vi "Data Recorder.vi"() -> ()   [LabVIEW 2017]
uses:
  LabVIEW/Controls/Recording Settings.ctl
  LabVIEW/Controls/Operator Settings.ctl
  LabVIEW/Controls/Operator.ctl
  LabVIEW/Controls/Patient Settings.ctl
  LabVIEW/Controls/Refnums.ctl
  LabVIEW/Controls/Dimensions.ctl
  LabVIEW/Controls/Room Dimensions.ctl
  LabVIEW/Controls/Crop Type.ctl
  <vilib>/vision/Image Controls.llb/IMAQ Image.ctl
  LabVIEW/Controls/Rigid Body Info.ctl
  LabVIEW/Controls/Position.ctl
  LabVIEW/Controls/Orientation.ctl
  LabVIEW/Controls/Enabled State Control.ctl
  LabVIEW/Controls/Frame Grabber State.ctl
  LabVIEW/Controls/Optitrack State.ctl
  LabVIEW/Controls/Frame Grabber Data.ctl
  <vilib>/userdefined/High Color/IMAQdx.ctl
  <vilib>/vision/Avi.llb/IMAQ AVI2 Refnum.ctl
  LabVIEW/Controls/Crop Video State.ctl
panel:
  out "Rigid Bodies":T1[](array[typedef])
  out "Mask":T4
  in  "Crop Type":T5
  out "Initial Recording Settings":T6={"Folder to Save Recordings"=path "", "Video FPS"=5, "Codec"=3, "Tracker FPS"=40, "Operator ID"={"Operator ID"=0, "Expertise"=0}, "Patient ID/Gestation"={"ID"=0, "Gestation"=""}} {"Patient ID/Gestation"."ID" format="%0#3.2f"; "Operator ID"."Operator ID" format="%03.0f"; "Operator ID"."Expertise" items=["Novice", "Expert"]; "Tracker FPS" max=100; "Codec" items=["Cinepak Codec by Radius", "Intel IYUV codec", "Microsoft Video 1", "FF Video Codec 1 (FFV1) (NI Vision)", "Motion JPEG (NI Vision)", "Y800 Uncompressed Grey Scale (NI Vision)", "YUV 4:2:0 Planar (NI Vision)"]; "Video FPS" max=100}
  in  "Dimensions":T10={"Probe Dimensions"={"Probe Width"=50.0, "Probe Depth"=100.0, "Probe Height"=150.0}, "Room Dimensions"={"Room Width"=1000.0, "Room Depth"=1000.0, "Room Height"=1000.0}}
  in  "Playback Rate":dbl(knob)=10.0 min=1.0 max=100.0 scale=1.0..100.0
  out "Time (s)":dbl caption="s"
  in  "Refnums":T12
  out "Tracked?":bool
  out "Crop ROI":i32[](array[numeric])
  in  "Clear Crop":bool
  in  "Append":bool
  in  "Presentation":string
  in  "Crop":bool
  in  "Pause":bool
  out "Video Playback Filename":path=path "C:/Users/lydia/Desktop/Images/Breech_Sacro_Posterior-20191119160600.avi"
  in  "Frame Slider":u32(slide)=175 scale=0.0..8635370.0
  in  "Playback":bool
  in  "Home":bool
  in  "Recording Settings":T6={"Folder to Save Recordings"=path "C:/Users/lydia/Desktop/Images", "Video FPS"=5, "Codec"=3, "Tracker FPS"=40, "Operator ID"={"Operator ID"=0, "Expertise"=0}, "Patient ID/Gestation"={"ID"=0, "Gestation"=""}} {"Patient ID/Gestation"."ID" format="%0#3.2f"; "Operator ID"."Operator ID" format="%03.0f"; "Operator ID"."Expertise" items=["Novice", "Expert"]; "Codec" items=["Cinepak Codec by Radius", "Intel IYUV codec", "Microsoft Video 1", "FF Video Codec 1 (FFV1) (NI Vision)", "Motion JPEG (NI Vision)", "Y800 Uncompressed Grey Scale (NI Vision)", "YUV 4:2:0 Planar (NI Vision)"]; "Video FPS" max=100}
  in  "Record":bool
  out "Tracker \nConnected?":bool
  out "Frame Grabber \nConnected?":bool
  out "Ultrasound Image":T4(plugin-control)
  in  "Live":bool
  in  "stop":bool
  in  "Probe Position":enum32{"3D", "Data"}(tab)
  out "Probe Position":refnum<vi>(3d-picture)
  out "Rigid Body":T1
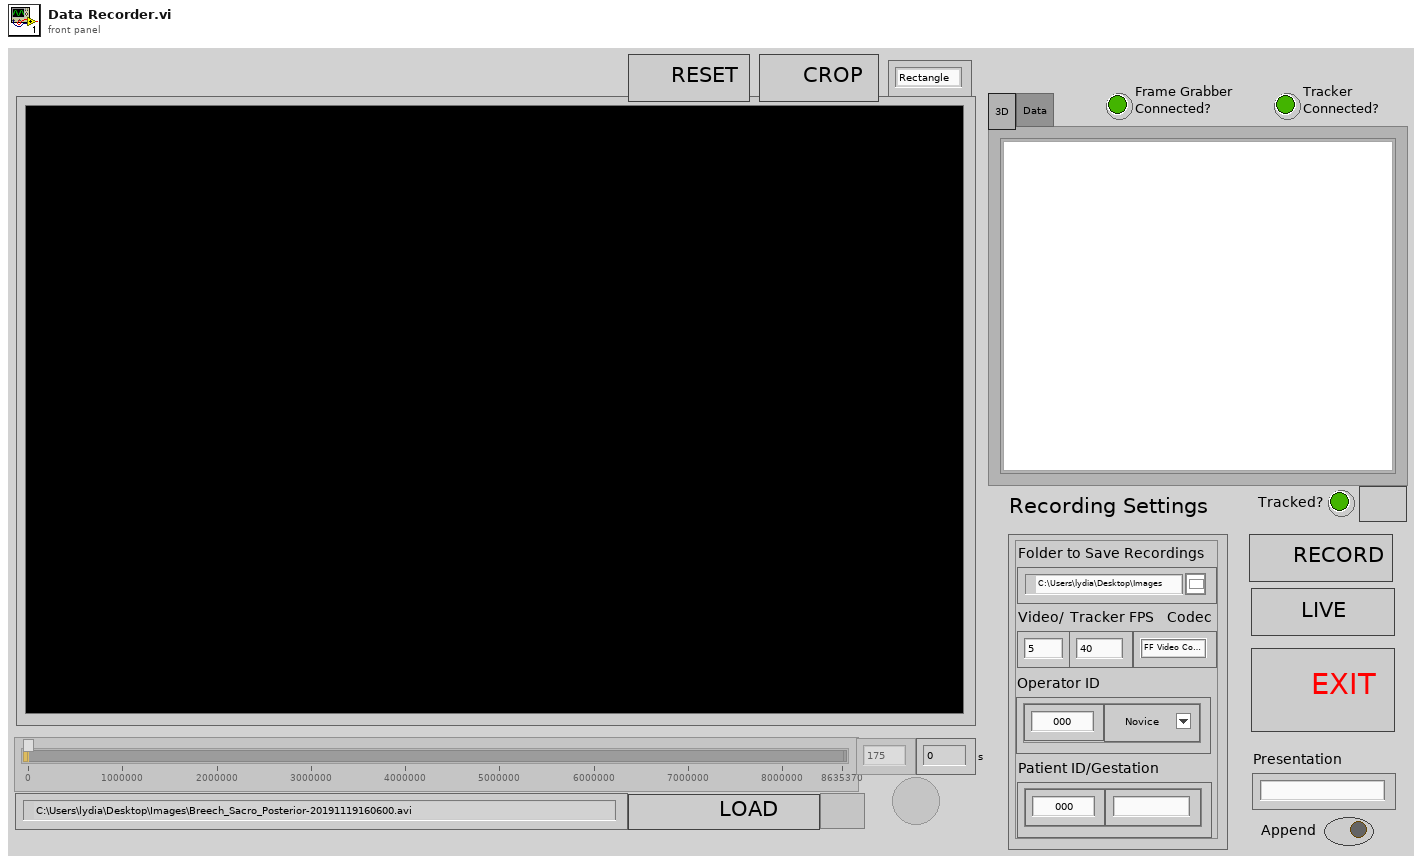
[diagram p1: front panel]
types:
  T1 = typedef "Rigid Body Info.ctl" = cluster{"Position":T2, "Orientation":T3, "Quaternion":cluster{"qx":sgl, "qy":sgl, "qz":sgl, "qw":sgl}, "Tracked?":bool}
  T2 = typedef "Position.ctl" = cluster{"x (mm)":sgl, "y (mm)":sgl, "z (mm)":sgl}
  T3 = typedef "Orientation.ctl" = cluster{"Pitch (rad)":sgl, "Yaw (rad)":sgl, "Roll (rad)":sgl}
  T4 = typedef "IMAQ Image.ctl" = refnum<image>
  T5 = typedef "Crop Type.ctl" = enum16{"Rectangle", "Annulus"}
  T6 = typedef "Recording Settings.ctl" = cluster{"Folder to Save Recordings":path, "Video FPS":u32, "Codec":u16, "Tracker FPS":u32, "Operator ID":T7, "Patient ID/Gestation":T9}
  T7 = typedef "Operator Settings.ctl" = cluster{"Operator ID":u32, "Expertise":T8}
  T8 = typedef "Operator.ctl" = u16
  T9 = typedef "Patient Settings.ctl" = cluster{"ID":u32, "Gestation":string}
  T10 = typedef "Dimensions.ctl" = cluster{"Probe Dimensions":cluster{"Probe Width":sgl, "Probe Depth":sgl, "Probe Height":sgl}, "Room Dimensions":T11}
  T11 = typedef "Room Dimensions.ctl" = cluster{"Room Width":dbl, "Room Depth":dbl, "Room Height":dbl}
  T12 = typedef "Refnums.ctl" = cluster{"Live Refnum":refnum<vi>, "Record Refnum":refnum<vi>, "Playback Refnum":refnum<vi>, "Frame Slider Refnum":refnum<vi>, "Pause Refnum":refnum<vi>, "Home Refnum":refnum<vi>, "Set Crop Refnum":refnum<vi>, "Clear Crop Refnum":refnum<vi>, "stop refnum":refnum<vi>, "Playback Rate Refnum":refnum<vi>, "Presentation Refnum":refnum<vi>, "Crop Time Frame Slider Refnum":refnum<vi>, "Cancel Save Refnum":refnum<vi>, "Reverse Playback Refnum":refnum<vi>, "Recording Settings Refnum":refnum<vi>, "Continuous Playback Refnum":refnum<vi>, "Annotation Refnum":refnum<vi>, "Export All Refnum":refnum<vi>, "Export List Refnum":refnum<vi>, "Fill List Refnum":refnum<vi>, "Save Crop Refnum":refnum<vi>, "Skip Forward Refnum":refnum<vi>, "Skip Backward Refnum":refnum<vi>, "Single Annotation Refnum":refnum<vi>, "Load Video Refnum":refnum<vi>, "Set Start Refnum":refnum<vi>, "Set End Refnum":refnum<vi>, "Add to List Refnum":refnum<vi>, "List of Annotations Refnum":refnum<vi>, "Camera Frame Refnum":refnum<vi>, "Load Image Refnum":refnum<vi>, "Saving Refnum":refnum<vi>}
  T13 = typedef "Enabled State Control.ctl" = enum16{"Init", "Wait", "Start Live", "Start Recording", "Start Playback", "Crop Set", "Crop Clear", "Shutdown"}
  T14 = typedef "Connection Settings.ctl" = cluster{"Frame Grabber":T15, "Tracker":T16, "Port":T17}
  T15 = typedef "IMAQdx.ctl" = refnum<k21>
  T16 = typedef "Tracker Type.ctl" = enum16{"Aurora", "OptiTrack"}
  T17 = typedef "COM Port.ctl" = enum16{"COM1", "COM2", "COM3", "COM4", "COM5", "COM6", "COM7", "COM8", "COM9", "COM10", "COM11", "COM12", "COM13", "COM14", "COM15", "COM16", "COM17", "COM18", "COM19", "COM20"}
  T18 = typedef "Frame Grabber Data.ctl" = cluster{"Camera Session":T15, "Frame":T4, "AVI Refnum":T19, "Codecs":string[], "Frame number":u32, "Tracking File Refnum":refnum<file>, "Tick Count":u32, "Probe Object":refnum<vi>, "Playback Probe Data":dbl[][], "Rigid Body":T1, "Total no frames playback":i32, "Video FPS":dbl, "Camera connected?":bool, "Scene":refnum<vi>, "Cropped Frame":T4, "Tracker FPS":dbl, "Crop ROI":i32[], "Presentation Values":string[], "Elapsed time (ms)":u32, "Camera frames playback":u32, "Refnums":T12, "Dimensions":T10, "Playback Data As Strings":string[][], "Cropped Tracking File Refnum":refnum<file>, "Cropped AVI Refnum":T19, "Header":string[], "Total euclidian distance":dbl, "Annotation File Path":path, "Playback File Path":path, "Size per frame":dbl, "Ground Truth File Refnum":refnum<file>, "Annotation Array":string[], "Annotation TIFFs Folder":path, "overwriting open file?":bool, "Image Sequence":T4[], "Video/Image Flag":T20, "Image sequence?":bool, "Image sequence filenames":string[], "Mask":T4, "Crop Type":T5}
  T19 = typedef "IMAQ AVI2 Refnum.ctl" = refnum<k20>
  T20 = typedef "Crop Video State.ctl" = enum16{"Init", "Wait", "Load Image", "Load Video", "Play/Pause", "Playback Video Frame", "Display Image", "Save Image Sequence", "Save Video", "Export List", "Export All", "Close", "Set Crop Area", "Reset Crop Area", "Crop Inside", "Crop Outside", "Multi-Crop", "Re-Open Files", "Annotate Frame", "Annotate Clip", "Add to List", "Fill List", "Set Start", "Set End", "Error Handling", "Shutdown"}
  T21 = typedef "Optitrack State.ctl" = enum16{"Wait", "Init", "Grab Rigid Body Data", "Error Handling", "Shutdown"}
  T22 = typedef "Frame Grabber State.ctl" = enum16{"Wait", "Init", "Update Geometry", "Set Crop ROI", "Clear Crop ROI", "Configure Live", "Configure Recording", "Start Playback", "Grab Live Frame", "Record Frame", "Playback Frame", "Unconfigure Live", "End Recording", "Stop Playback", "Error Handling", "Shutdown"}
  T23 = typedef "Queues.ctl" = cluster{"Frame Grabber State":refnum<queue>, "Tracker State":refnum<queue>, "Frame Number Semaphore":T24}
  T24 = typedef "Semaphore RefNum" = refnum<k1>
  T25 = enum8{"Enabled", "Disabled", "Disabled and Grayed Out"}
  T26 = typedef "Tracking Data.ctl" = cluster{"VISA resource name":refnum<visa-resource-name>, "Packet Data":T27, "Rigid Body Data":T1[], "Position Array":dbl[][], "Tracker":T16, "Number of Tools":u32}
  T27 = typedef "Packet Data.ctl" = cluster{"Frame Number (UINT32)":u32, "Number of Rigid Bodies (UINT32)":u32, "Timestamp (double float)":dbl}
  T28 = typedef "Tracking Data Multi Body.ctl" = cluster{"VISA resource name":refnum<visa-resource-name>, "Packet Data":T27, "Rigid Body Data":T1[], "Position Array":dbl[][], "Tracker":T16, "Number of Tools":u32}
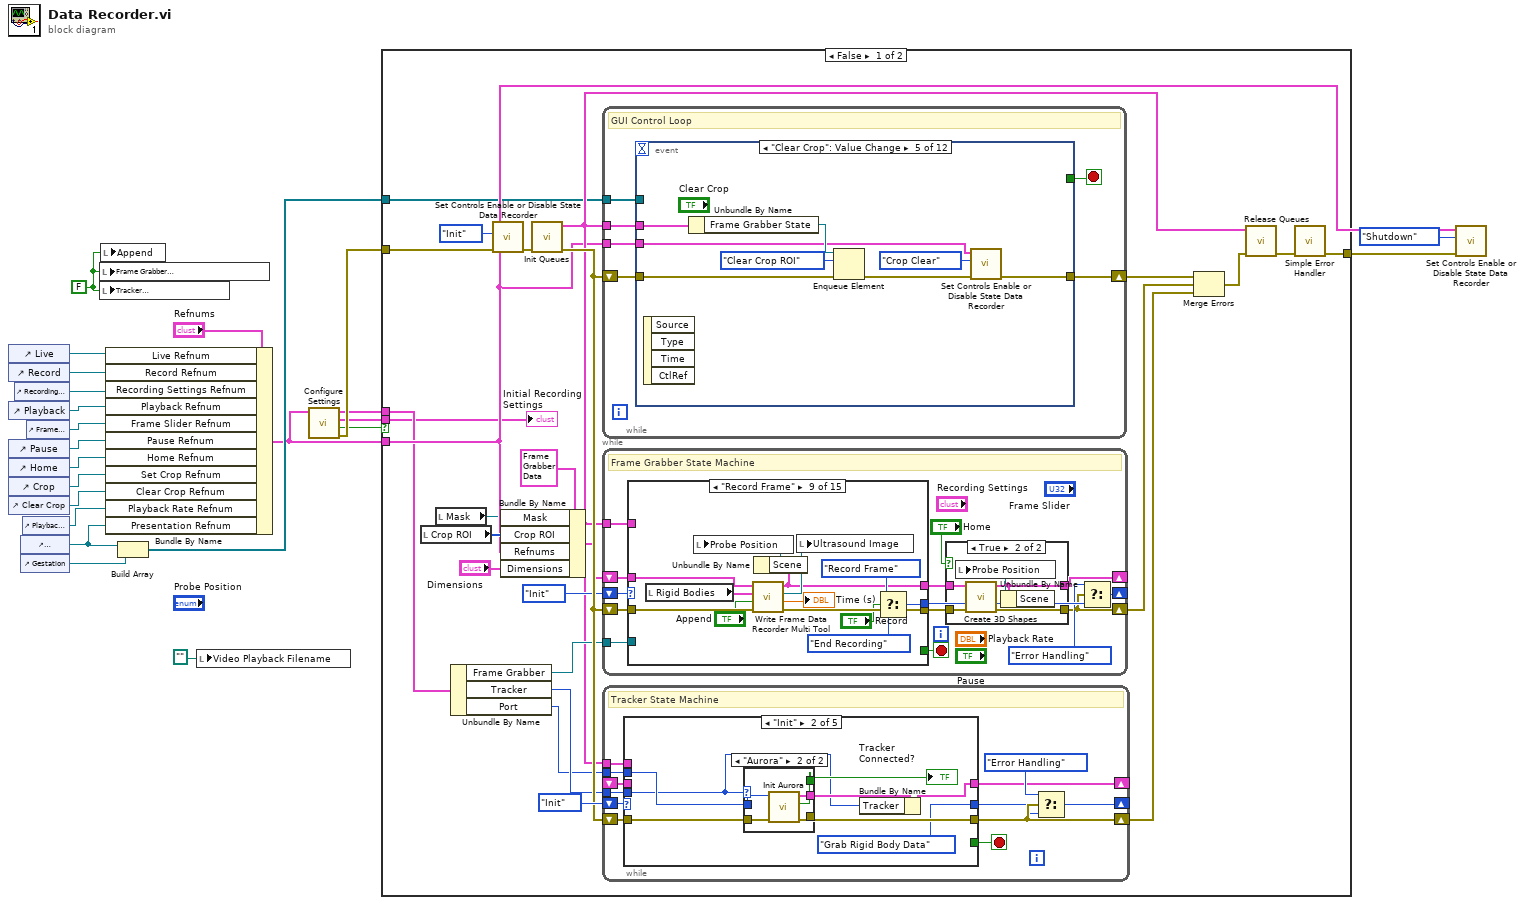
[diagram p0: block diagram]
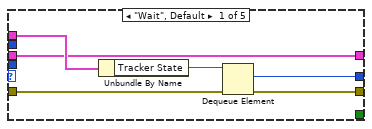
[diagram p2: hidden frame]
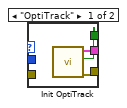
[diagram p3: hidden frame]
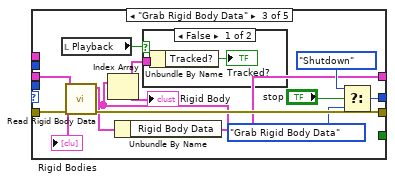
[diagram p4: hidden frame]
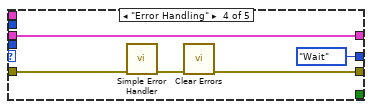
[diagram p6: hidden frame]
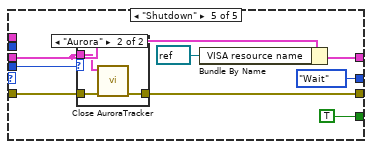
[diagram p7: hidden frame]
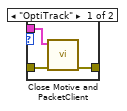
[diagram p8: hidden frame]
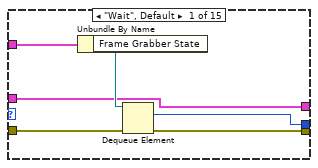
[diagram p10: hidden frame]
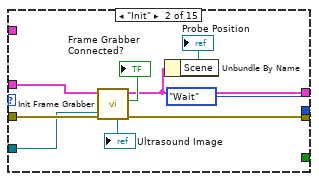
[diagram p11: hidden frame]
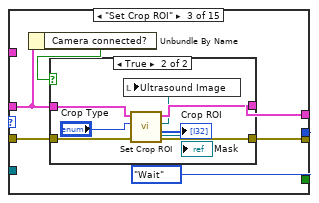
[diagram p12: hidden frame]
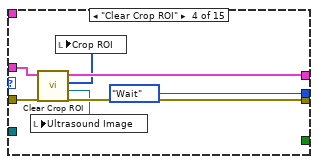
[diagram p14: hidden frame]
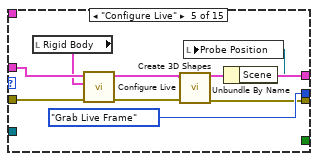
[diagram p15: hidden frame]
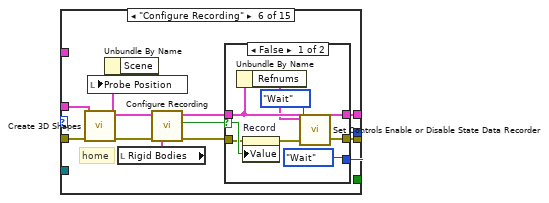
[diagram p16: hidden frame]
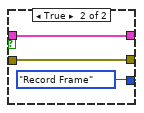
[diagram p17: hidden frame]
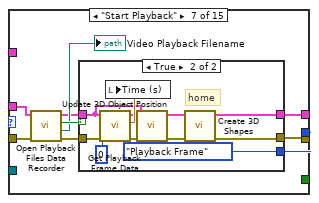
[diagram p18: hidden frame]
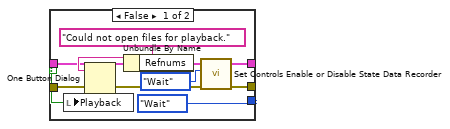
[diagram p19: hidden frame]
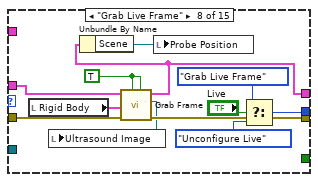
[diagram p20: hidden frame]
diagram:
  w14 = FALSE ("Camera Connected?")
  n1 = control-ref of="Live"() -> (w23:refnum<vi>)
  n2 = control-ref of="Record"() -> (w22:refnum<vi>)
  n3 = control-ref of="Playback"() -> (w21:refnum<vi>)
  n4 = control-ref of="Pause"() -> (w19:refnum<vi>)
  n5 = control-ref of="Home"() -> (w18:refnum<vi>)
  n6 = control-ref of="Crop"() -> (w17:refnum<vi>)
  n7 = control-ref of="Clear Crop"() -> (w16:refnum<vi>)
  n8 = control-ref of="Recording Settings"() -> (w6:refnum<vi>)
  n9 = control-ref of="Presentation"() -> (w11:refnum<vi>)
  n10 = control-ref of="Gestation"() -> (w5:refnum<vi>)
  n11 = control-ref of="Playback Rate"() -> (w12:refnum<vi>)
  n12 = control-ref of="Frame Slider"() -> (w20:refnum<vi>)
  n13 = local write "Frame Grabber \nConnected?"(w14) -> ()
  n14 = local write "Tracker \nConnected?"(w14) -> ()
  n15 = local write "Append"(w14) -> ()
  n16 = Bundle By Name(cluster="Refnums", "Live Refnum"=w23, "Record Refnum"=w22, "Recording Settings Refnum"=w6, "Playback Refnum"=w21, "Frame Slider Refnum"=w20, "Pause Refnum"=w19, "Home Refnum"=w18, "Set Crop Refnum"=w17, "Clear Crop Refnum"=w16, "Playback Rate Refnum"=w12, "Presentation Refnum"=w11) -> (w7:T12)
  n17 = Build Array(w11, w5) -> (w10:refnum<vi>[])
  n18 = local write "Video Playback Filename"(path "") -> ()
  n19 = call "Configure Settings.vi"("Refnums"=w7) -> ("Error Out"=w9:errorcluster, "Cancelled?"=w3:bool, "Recording Settings Out"=w2:T6, "Connection Settings Out"=w8:T14)  [unwired: 7 in]
  n20 = case shown="False" w3 {
    tunnel: [w38 w462] -> w13
    tunnel: w10 -> [w29 _]
    tunnel: w9 -> [w28 w462]
    tunnel: w8 -> [w27 _]
    tunnel: w7 -> [w26 _]
    tunnel: w2 -> [w25 _]
    frame False {
      n21 = local read "Crop ROI"() -> (w30:i32[])
      n22 = local read "Mask"() -> (w24:T4)
      n23 = Unbundle By Name(w27) -> ("Frame Grabber"=w37:T15, "Tracker"=w36:T16, "Port"=w35:T17)
      n24 = call "Set Controls Enable or Disable State Data Recorder.vi"("error in (no error)"=w28, "Refnum State"=Enabled_State_Control."Init", "Refnums In"=w26) -> ("error out"=w40:errorcluster)  [unwired: 8 in]
      n25 = Bundle By Name(cluster=T18 {"Camera Session"="", "Frame"=refnum, "AVI Refnum"=refnum, "Codecs"=[], "Frame number"=0, "Tracking File Refnum"=refnum, "Tick Count"=0, "Probe Object"=refnum, "Playback Probe Data"=[], "Rigid Body"={"Position"={"x (mm)"=0.0, "y (mm)"=0.0, "z (mm)"=0.0}, "Orientation"={"Pitch (rad)"=0.0, "Yaw (rad)"=0.0, "Roll (rad)"=0.0}, "Quaternion"={"qx"=0.0, "qy"=0.0, "qz"=0.0, "qw"=0.0}, "Tracked?"=FALSE}, "Total no frames playback"=0, "Video FPS"=0.0, "Camera connected?"=FALSE, "Scene"=refnum, "Cropped Frame"=refnum, "Tracker FPS"=0.0, "Crop ROI"=[], "Presentation Values"=[], "Elapsed time (ms)"=0, "Camera frames playback"=0, "Refnums"={"Live Refnum"=refnum, "Record Refnum"=refnum, "Playback Refnum"=refnum, "Frame Slider Refnum"=refnum, "Pause Refnum"=refnum, "Home Refnum"=refnum, "Set Crop Refnum"=refnum, "Clear Crop Refnum"=refnum, "stop refnum"=refnum, "Playback Rate Refnum"=refnum, "Presentation Refnum"=refnum, "Crop Time Frame Slider Refnum"=refnum, "Cancel Save Refnum"=refnum, "Reverse Playback Refnum"=refnum, "Recording Settings Refnum"=refnum, "Continuous Playback Refnum"=refnum, "Annotation Refnum"=refnum, "Export All Refnum"=refnum, "Export List Refnum"=refnum, "Fill List Refnum"=refnum, "Save Crop Refnum"=refnum, "Skip Forward Refnum"=refnum, "Skip Backward Refnum"=refnum, "Single Annotation Refnum"=refnum, "Load Video Refnum"=refnum, "Set Start Refnum"=refnum, "Set End Refnum"=refnum, "Add to List Refnum"=refnum, "List of Annotations Refnum"=refnum, "Camera Frame Refnum"=refnum, "Load Image Refnum"=refnum, "Saving Refnum"=refnum}, "Dimensions"={"Probe Dimensions"={"Probe Width"=0.0, "Probe Depth"=1.0, "Probe Height"=0.0}, "Room Dimensions"={"Room Width"=0.0, "Room Depth"=0.0, "Room Height"=0.0}}, "Playback Data As Strings"=[], "Cropped Tracking File Refnum"=refnum, "Cropped AVI Refnum"=refnum, "Header"=[], "Total euclidian distance"=0.0, "Annotation File Path"=path "", "Playback File Path"=path "", "Size per frame"=0.0, "Ground Truth File Refnum"=refnum, "Annotation Array"=[], "Annotation TIFFs Folder"=path "", "overwriting open file?"=FALSE, "Image Sequence"=[], "Video/Image Flag"=enum."Playback Video Frame", "Image sequence?"=FALSE, "Image sequence filenames"=[], "Mask"=refnum, "Crop Type"=enum."Rectangle"} ("Frame Grabber Data out"), "Mask"=w24, "Crop ROI"=w30, "Refnums"=w26, "Dimensions"="Dimensions") -> (w34:T18)
      n26 = call "Init Queues.vi"("error in (no error) in"=w40) -> ("error out"=w43:errorcluster, "Queues"=w32:T23)  [unwired: 9 in]
      n27 = while {
        shift-right: [w330] -> w48
        shift-left: w43 -> [w331]
        tunnel: w32 -> [w329]
        tunnel: w26 -> [w328]
        tunnel: w29 -> [w327]
        stop <- w332 stop-if-true
        # "GUI Control Loop"
        n28 = event shown="[4] \"Clear Crop\": Value Change" {
          selector: _ -> [_ _ _ _ _ _ _ _ _ _ _ _]
          dyn-events: _ -> [_ _ _ _ _ _ _ _ _ _ _ _]
          timeout: _ -> [_ _ _ _ _ _ _ _ _ _ _ _]
          tunnel: [w335 _ _ _ _ _ _ _ _ _ _ _] -> w332
          tunnel: w331 -> [w334 w355 w369 w377 w385 w398 w399 w413 w416 w424 w434 w460]
          tunnel: [w338 w348 w360 w372 w379 w389 w399 w411 w416 w420 w435 w460] -> w330
          tunnel: w329 -> [w342 w352 w366 w376 w384 w395 _ _ _ w418 _ _]
          tunnel: w328 -> [_ w347 w362 w371 w378 w391 _ _ _ _ _ _]
          tunnel: w327 -> [_ _ _ _ _ _ _ _ _ _ w430 _]
          event "stop": Value Change {
            w333 = FALSE ("Run")
            n29 = event-data() -> ("NewVal"=w335:bool)  [unwired: 1 in]
            n30 = local write "Tracker \nConnected?"(w333) -> ()
            n31 = local write "Append"(w333) -> ()
            n32 = local write "Frame Grabber \nConnected?"(w333) -> ()
            n33 = local write "Live"(w333) -> ()
            n34 = local write "Record"(w333) -> ()
            n35 = local write "Pause"(w333) -> ()
            n36 = Unbundle By Name(w342) -> ("Tracker State"=w337:refnum<queue>, "Frame Grabber State"=w341:refnum<queue>)
            n37 = local write "Playback"(w333) -> ()
            n38 = Enqueue Element(queue=w341, element=Frame_Grabber_State."Shutdown", error in (no error)=w334) -> (error out=w339:errorcluster)  [unwired: 1 in, 2 out]
            n39 = Enqueue Element(queue=w337, element=Optitrack_State."Shutdown", error in (no error)=w339) -> (error out=w338:errorcluster)  [unwired: 1 in, 2 out]
          }
          event "Live": Value Change {
            n40 = event-data() -> ("NewVal"=w344:bool)  [unwired: 1 in]
            n41 = Unbundle By Name(w352) -> ("Frame Grabber State"=w351:refnum<queue>)
            n42 = Select(t=Frame_Grabber_State."Configure Live", s=w344, f=Frame_Grabber_State."Wait") -> (s? t:f=w353:T22)
            n43 = Enqueue Element(queue=w351, element=w353, error in (no error)=w355) -> (error out=w349:errorcluster)  [unwired: 1 in, 2 out]
            n44 = Select(t=Enabled_State_Control."Start Live" ("Refnum State"), s=w344, f=Enabled_State_Control."Wait") -> (s? t:f=w345:T13)
            n45 = call "Set Controls Enable or Disable State Data Recorder.vi"("error in (no error)"=w349, "Refnum State"=w345, "Refnums In"=w347) -> ("error out"=w348:errorcluster)  [unwired: 8 in]
          }
          event "Playback": Value Change {
            n46 = event-data() -> ("NewVal"=w358:bool)  [unwired: 1 in]
            n47 = Unbundle By Name(w366) -> ("Frame Grabber State"=w365:refnum<queue>)
            n48 = Select(t=Frame_Grabber_State."Start Playback", s=w358, f=Frame_Grabber_State."Wait") -> (s? t:f=w367:T22)
            n49 = Enqueue Element(queue=w365, element=w367, error in (no error)=w369) -> (error out=w361:errorcluster)  [unwired: 1 in, 2 out]
            n50 = Select(t=Enabled_State_Control."Start Playback", s=w358, f=Enabled_State_Control."Wait" ("Refnum State")) -> (s? t:f=w357:T13)
            n51 = local write "Pause"(FALSE ("Pause")) -> ()
            n52 = call "Set Controls Enable or Disable State Data Recorder.vi"("error in (no error)"=w361, "Refnum State"=w357, "Refnums In"=w362) -> ("error out"=w360:errorcluster)  [unwired: 8 in]
          }
          event "Crop": Value Change {
            n53 = event-data() -> ()  [unwired: 1 in, 4 out]
            n54 = Unbundle By Name(w376) -> ("Frame Grabber State"=w375:refnum<queue>)
            n55 = Enqueue Element(queue=w375, element=Frame_Grabber_State."Set Crop ROI", error in (no error)=w377) -> (error out=w373:errorcluster)  [unwired: 1 in, 2 out]
            n56 = call "Set Controls Enable or Disable State Data Recorder.vi"("error in (no error)"=w373, "Refnum State"=Enabled_State_Control."Crop Set", "Refnums In"=w371) -> ("error out"=w372:errorcluster)  [unwired: 8 in]
          }
          event "Clear Crop": Value Change {
            n57 = event-data() -> ()  [unwired: 1 in, 4 out]
            n58 = Unbundle By Name(w384) -> ("Frame Grabber State"=w383:refnum<queue>)
            n59 = Enqueue Element(queue=w383, element=Frame_Grabber_State."Clear Crop ROI", error in (no error)=w385) -> (error out=w380:errorcluster)  [unwired: 1 in, 2 out]
            n60 = call "Set Controls Enable or Disable State Data Recorder.vi"("error in (no error)"=w380, "Refnum State"=Enabled_State_Control."Crop Clear", "Refnums In"=w378) -> ("error out"=w379:errorcluster)  [unwired: 8 in]
          }
          event "Record": Value Change {
            n61 = event-data() -> ("NewVal"=w392:bool)  [unwired: 1 in]
            n62 = Unbundle By Name(w395) -> ("Frame Grabber State"=w394:refnum<queue>)
            n63 = Select(t=Frame_Grabber_State."Configure Recording", s=w392, f=Frame_Grabber_State."Wait") -> (s? t:f=w396:T22)
            n64 = Enqueue Element(queue=w394, element=w396, error in (no error)=w398) -> (error out=w390:errorcluster)  [unwired: 1 in, 2 out]
            n65 = Select(t=Enabled_State_Control."Start Recording" ("Refnum State"), s=w392, f=Enabled_State_Control."Wait" ("Refnum State")) -> (s? t:f=w386:T13)
            n66 = call "Set Controls Enable or Disable State Data Recorder.vi"("error in (no error)"=w390, "Refnum State"=w386, "Refnums In"=w391) -> ("error out"=w389:errorcluster)  [unwired: 8 in]
          }
          event "Presentation": Value Change {
            n67 = event-data() -> ()  [unwired: 1 in, 1 out]
            n68 = local write "Append"(TRUE ("Append")) -> ()
          }
          event Value Change {
            w405 = "_"
            # "remove spaces and periods"
            n69 = event-data() -> ("CtlRef"=w414:refnum<vi>)  [unwired: 1 in, 2 out]
            n70 = property class="Str"(reference=w414, error in=w413) -> (reference out=w412:refnum<vi>, error out=w408:errorcluster, "Value"=w410:string)
            n71 = call <vilib>:"Space Constant.vi"() -> ("String"=w409:string)
            n72 = Search and Replace String(replace all?=TRUE ("replace all? (F)"), input string=w410, search string=w409, replace string=w405, error in=w408) -> (result string=w404:string, error out=w403:errorcluster)  [unwired: 3 in, 2 out]
            n73 = Search and Replace String(replace all?=TRUE ("replace all? (F)"), input string=w404, search string=".", replace string=w405, error in=w403) -> (error out=w402:errorcluster)  [unwired: 3 in, 3 out]
            n74 = property class="Str"(reference=w412, error in=w402, "Value"=w404) -> (error out=w411:errorcluster)  [unwired: 1 out]
          }
          event Value Change {
            n75 = event-data() -> ("NewVal"=w415:T6)  [unwired: 1 in]
            n76 = local write "Initial Recording Settings"(w415) -> ()
          }
          event "Frame Slider": Value Change {
            n77 = event-data() -> ()  [unwired: 1 in, 1 out]
            n78 = Unbundle By Name(w418) -> ("Frame Number Semaphore"=w417:T24)
            n79 = call <vilib>:"Acquire Semaphore.vi"("error in (no error)"=w424, "semaphore"=w417) -> ("error out"=w421:errorcluster, "timed out"=w423:bool, "semaphore out"=w419:T24)  [unwired: 3 in]
            n80 = case shown="False" w423 {
              tunnel: [w425 w427] -> w422
              tunnel: w421 -> [w425 w427]
              frame False {
                n81 = Wait (ms)(milliseconds to wait=u32 50) -> ()  [unwired: 1 out]
              }
              frame True {
              }
            }
            n82 = call <vilib>:"Release Semaphore.vi"("error in (no error)"=w422, "semaphore"=w419) -> ("error out"=w420:errorcluster)  [unwired: 4 in, 1 out]
          }
          event Key Down {
            n83 = event-data() -> ("FocusObj"=w431:refnum<vi>, "Char"=w436:i16)  [unwired: 1 in]
            n84 = property on="Pause" class="Bool (strict)"(error in=w434) -> (error out=w433:errorcluster, "DisabledEnum"=w432:T25)  [unwired: 1 in, 1 out]
            n85 = Equal?(x=w430, y=w431) -> (x = y?=w429:bool[])
            n86 = Or Array Elements(Boolean array=w429) -> (logical OR=w428:bool)
            n87 = case shown="\"Enabled\"" w432 {
              tunnel: w436 -> [_ w441]
              tunnel: [w437 w440] -> w435
              tunnel: w433 -> [w437 w439]
              tunnel: w428 -> [_ w438]
              frame Default {
              }
              frame "Enabled" {
                n88 = case shown="False" w438 {
                  tunnel: w441 -> [w444 _]
                  tunnel: [w443 w455] -> w440
                  tunnel: w439 -> [w442 w455]
                  frame False {
                    # "space bar controls \nplay toggle"
                    n89 = Type Cast(type="", x=w444) -> (*(type *) &x=w448:string)
                    n90 = String Subset(string=w448, offset (0)=1) -> (substring=w445:string)  [unwired: 1 in]
                    n91 = case shown="\" \"" w445 {
                      tunnel: w442 -> [w449 w454]
                      tunnel: [w449 w452] -> w443
                      frame Default {
                        # "do nothing"
                      }
                      frame " " {
                        # "toggle"
                        n92 = property on="Pause" class="Bool (strict)"(error in=w454) -> (error out=w453:errorcluster, "Value"=w451:bool)  [unwired: 1 in, 1 out]
                        n93 = Not(x=w451) -> (.not. x?=w450:bool)
                        n94 = property on="Pause" class="Bool (strict)"(error in=w453, "Value"=w450) -> (error out=w452:errorcluster)  [unwired: 1 in, 1 out]
                      }
                    }
                  }
                  frame True {
                  }
                }
              }
            }
          }
          event Value Change {
            n95 = event-data() -> ()  [unwired: 1 in, 3 out]
            n96 = local read "Recording Settings"() -> (w459:T6)
            n97 = Unbundle By Name(w459) -> ("Video FPS"=w458:u32, "Tracker FPS"=w457:u32)
            n98 = Greater?(x=w458, y=w457) -> (0:w456:bool)
            n99 = case shown="False" w456 {
              frame False {
              }
              frame True {
                n100 = One Button Dialog(message="Warning! Unexpected behaviour if frame grabber recording rate is higher than tracker recording rate.") -> ()  [unwired: 1 in, 1 out]
              }
            }
          }
        }
      }
      n101 = while {
        shift-right: [w123] -> _
        shift-left: Frame_Grabber_State."Init" -> [w128]
        shift-right: [w118] -> w47
        shift-left: w43 -> [w127]
        shift-right: [w116] -> _
        shift-left: w34 -> [w125]
        tunnel: w37 -> [w121]
        tunnel: w32 -> [w120]
        stop <- w126 stop-if-true
        # "Frame Grabber State Machine"
        n102 = case shown="\"Record Frame\"" w128 {
          tunnel: w127 -> [w141 w150 w155 w171 w182 w193 w214 w245 w255 w266 w291 w295 w309 w316 w324]
          tunnel: [w140 w147 w154 w170 w177 w187 w211 w244 w254 w262 w289 w292 w299 w313 w323] -> w119
          tunnel: [w138 Frame_Grabber_State."Wait" Frame_Grabber_State."Wait" Frame_Grabber_State."Wait" Frame_Grabber_State."Grab Live Frame" w194 w210 w242 w256 w277 Frame_Grabber_State."Wait" Frame_Grabber_State."Wait" Frame_Grabber_State."Wait" Frame_Grabber_State."Wait" Frame_Grabber_State."Wait"] -> w124
          tunnel: [_ _ _ _ _ _ _ _ _ _ _ _ _ _ TRUE] -> w126
          tunnel: [w137 w143 w153 w169 w175 w184 w206 w238 w249 w272 w288 w293 w306 w311 w321] -> w117
          tunnel: w125 -> [w137 w144 w152 w172 w181 w192 w213 w241 w251 w273 w288 w293 w307 w311 w322]
          tunnel: w121 -> [_ w145 _ _ _ _ _ _ _ _ _ _ _ _ _]
          tunnel: w120 -> [w136 _ _ _ _ _ _ _ _ w260 _ _ _ _ _]
          frame "Wait", Default {
            n103 = Unbundle By Name(w136) -> ("Frame Grabber State"=w139:refnum<queue>)
            n104 = Dequeue Element(queue=w139, error in (no error)=w141) -> (element=w138:T22, error out=w140:errorcluster)  [unwired: 1 in, 2 out]
          }
          frame "Init" {
            n105 = call "Init Frame Grabber.vi"("Frame Grabber"=w145, "Error In"=w150, "Frame Grabber Data In"=w144) -> ("Error Out"=w147:errorcluster, "Frame Grabber Connected?"=→"Frame Grabber \nConnected?":bool, "Frame Grabber Data Out"=w143:T18, "Image Out"=→"Ultrasound Image":T4)  [unwired: 5 in]
            n106 = Unbundle By Name(w143) -> ("Scene"=→"Probe Position":refnum<vi>)
          }
          frame "Set Crop ROI" {
            n107 = Unbundle By Name(w152) -> ("Camera connected?"=w151:bool)
            n108 = case shown="True" w151 {
              tunnel: w155 -> [w158 w166]
              tunnel: [w158 w165] -> w154
              tunnel: w152 -> [w157 w164]
              tunnel: [w157 w163] -> w153
              frame False {
                # "don't crop, no image\nto crop!"
              }
              frame True {
                n109 = call "Set Crop ROI.vi"("error in (no error)"=w166, "Crop Type"="Crop Type", "Frame Grabber Data in"=w164) -> ("error out"=w165:errorcluster, "Crop ROI"=→"Crop ROI":i32[], "Image Out"=w162:T4, "Frame Grabber Data out"=w163:T18, "mask"=→"Mask":T4)  [unwired: 3 in, 1 out]
                n110 = local write "Ultrasound Image"(w162) -> ()
              }
            }
          }
          frame "Clear Crop ROI" {
            n111 = call "Clear Crop ROI.vi"("error in (no error)"=w171, "Frame Grabber Data in"=w172) -> ("error out"=w170:errorcluster, "Image Out"=w168:T4, "Crop ROI"=w167:i32[], "Frame Grabber Data out"=w169:T18)  [unwired: 6 in]
            n112 = local write "Ultrasound Image"(w168) -> ()
            n113 = local write "Crop ROI"(w167) -> ()
          }
          frame "Configure Live" {
            n114 = local read "Rigid Body"() -> (w179:T1)
            n115 = call "Configure Live.vi"("error in (no error)"=w182, "Rigid Body"=w179, "Frame Grabber Data in"=w181) -> ("error out"=w178:errorcluster, "Frame Grabber Data out"=w176:T18)  [unwired: 7 in]
            n116 = call "Create 3D Shapes.vi"("error in (no error)"=w178, "Frame Grabber Data In"=w176) -> ("error out"=w177:errorcluster, "Frame Grabber Data Out"=w175:T18)  [unwired: 8 in]
            n117 = Unbundle By Name(w175) -> ("Scene"=w174:refnum<vi>)
            n118 = local write "Probe Position"(w174) -> ()
          }
          frame "Configure Recording" {
            # "home"
            n119 = call "Create 3D Shapes.vi"("error in (no error)"=w193, "Frame Grabber Data In"=w192) -> ("error out"=w188:errorcluster, "Frame Grabber Data Out"=w191:T18)  [unwired: 8 in]
            n120 = Unbundle By Name(w191) -> ("Scene"=w190:refnum<vi>)
            n121 = local write "Probe Position"(w190) -> ()
            n122 = local read "Rigid Bodies"() -> (w189:T1[])
            n123 = call "Configure Recording.vi"("error in (no error)"=w188, "Rigid Bodies"=w189, "Frame Grabber Data In"=w191) -> ("error out"=w183:errorcluster, "Record?"=w186:bool, "Frame Grabber Data Out"=w185:T18)  [unwired: 6 in]
            n124 = case shown="False" w186 {
              selector: w186 -> [w196 _]
              tunnel: [Frame_Grabber_State."Wait" Frame_Grabber_State."Record Frame"] -> w194
              tunnel: [w198 w203] -> w184
              tunnel: [w200 w204] -> w187
              tunnel: w185 -> [w198 w203]
              tunnel: w183 -> [w195 w204]
              frame False {
                n125 = Unbundle By Name(w198) -> ("Refnums"=w197:T12)
                n126 = property on="Record" class="Bool (strict)"(error in=w195, "Value"=w196) -> (error out=w201:errorcluster)  [unwired: 1 in, 1 out]
                n127 = call "Set Controls Enable or Disable State Data Recorder.vi"("error in (no error)"=w201, "Refnum State"=Enabled_State_Control."Wait", "Refnums In"=w197) -> ("error out"=w200:errorcluster)  [unwired: 8 in]
              }
              frame True {
              }
            }
          }
          frame "Start Playback" {
            n128 = call "Open Playback Files Data Recorder.vi"("error in (no error)"=w214, "Frame Grabber Data In"=w213) -> ("error out"=w212:errorcluster, "Playback Video"=→"Video Playback Filename":path, "both exist and open?"=w209:bool, "Frame Grabber Data Out"=w207:T18)  [unwired: 6 in]
            n129 = case shown="True" w209 {
              selector: w209 -> [w220 _]
              tunnel: w212 -> [w219 w232]
              tunnel: [w218 w231] -> w211
              tunnel: [Frame_Grabber_State."Wait" ("f") Frame_Grabber_State."Playback Frame"] -> w210
              tunnel: w207 -> [w216 w225]
              tunnel: [w216 w227] -> w206
              frame False {
                n130 = local write "Playback"(w220) -> ()
                n131 = One Button Dialog(message="Could not open files for playback.") -> ()  [unwired: 1 in, 1 out]
                n132 = Unbundle By Name(w216) -> ("Refnums"=w215:T12)
                n133 = call "Set Controls Enable or Disable State Data Recorder.vi"("error in (no error)"=w219, "Refnum State"=Enabled_State_Control."Wait", "Refnums In"=w215) -> ("error out"=w218:errorcluster)  [unwired: 8 in]
              }
              frame True {
                # "home"
                n134 = call "Get Playback Frame Data.vi"("Error In"=w232, "Frame number"=u32 0, "Frame Grabber Data"=w225) -> ("Error Out"=w224:errorcluster, "Time elapsed (s)"=w229:dbl, "New Rigid Body Position"=w226:T1)  [unwired: 4 in, 2 out]
                n135 = local write "Time (s)"(w229) -> ()
                n136 = call "Update 3D Object Position.vi"("error in (no error)"=w224, "New Rigid Body Position"=w226, "Frame Grabber Data in"=w225) -> ("error out"=w228:errorcluster, "Frame Grabber Data out"=w223:T18)  [unwired: 7 in]
                n137 = call "Create 3D Shapes.vi"("error in (no error)"=w228, "Frame Grabber Data In"=w223) -> ("error out"=w231:errorcluster, "Frame Grabber Data Out"=w227:T18)  [unwired: 8 in]
              }
            }
          }
          frame "Grab Live Frame" {
            w236 = TRUE
            n138 = local read "Rigid Body"() -> (w240:T1)
            n139 = call "Grab Frame.vi"("Live?"=w236, "Grab frame?"=w236, "error in (no error)"=w245, "Rigid Body"=w240, "Frame Grabber Data in"=w241) -> ("error out"=w244:errorcluster, "Frame"=w235:T4, "Frame Grabber Data out"=w238:T18)  [unwired: 3 in, 1 out]
            n140 = local write "Ultrasound Image"(w235) -> ()
            n141 = Unbundle By Name(w238) -> ("Scene"=w239:refnum<vi>)
            n142 = local write "Probe Position"(w239) -> ()
            n143 = Select(t=Frame_Grabber_State."Grab Live Frame", s="Live", f=Frame_Grabber_State."Unconfigure Live") -> (s? t:f=w242:T22)
          }
          frame "Record Frame" {
            n144 = local read "Rigid Bodies"() -> (w253:T1[])
            n145 = call "Write Frame Data Recorder Multi Tool.vi"("error in (no error)"=w255, "Append"="Append", "Rigid Bodies"=w253, "Frame Grabber Data In in"=w251) -> ("error out"=w254:errorcluster, "Time elapsed (s)"=→"Time (s)":dbl, "Image"=w252:T4, "Frame Grabber Data out"=w249:T18)  [unwired: 2 in, 2 out]
            n146 = Unbundle By Name(w249) -> ("Scene"=w250:refnum<vi>)
            n147 = local write "Probe Position"(w250) -> ()
            n148 = local write "Ultrasound Image"(w252) -> ()
            n149 = Select(t=Frame_Grabber_State."Record Frame", s="Record", f=Frame_Grabber_State."End Recording") -> (s? t:f=w256:T22)
          }
          frame "Playback Frame" {
            n150 = Unbundle By Name(w260) -> ("Frame Number Semaphore"=w259:T24)
            n151 = call <vilib>:"Acquire Semaphore.vi"("error in (no error)"=w266, "semaphore"=w259) -> ("error out"=w265:errorcluster, "timed out"=w264:bool, "semaphore out"=w261:T24)  [unwired: 3 in]
            n152 = case shown="False" w264 {
              tunnel: w273 -> [w285 w286]
              tunnel: [w284 w286] -> w272
              tunnel: [w283 _] -> w270
              tunnel: [w282 w287] -> w263
              tunnel: [w281 _] -> w269
              tunnel: [w280 _] -> w267
              tunnel: w265 -> [w279 w287]
              frame False {
                n153 = call "Playback Frame Data Recorder.vi"("error in (no error)"=w279, "Frame Grabber Data in"=w285) -> ("error out"=w282:errorcluster, "Continue playback?"=w281:bool, "Image"=w280:T4, "Frame Grabber Data out"=w284:T18, "Time elapsed (s)"=w283:dbl)  [unwired: 5 in]
              }
              frame True {
              }
            }
            n154 = Unbundle By Name(w272) -> ("Rigid Body.Tracked?"=w268:bool, "Scene"=w271:refnum<vi>)
            n155 = local write "Time (s)"(w270) -> ()
            n156 = call <vilib>:"Release Semaphore.vi"("error in (no error)"=w263, "semaphore"=w261) -> ("error out"=w262:errorcluster)  [unwired: 4 in, 1 out]
            n157 = local write "Tracked?"(w268) -> ()
            n158 = local write "Probe Position"(w271) -> ()
            n159 = local write "Ultrasound Image"(w267) -> ()
            n160 = And(x=w269, y="Playback") -> (x .and. y?=w275:bool)
            n161 = Select(t=Frame_Grabber_State."Playback Frame", s=w275, f=Frame_Grabber_State."Stop Playback") -> (s? t:f=w277:T22)
          }
          frame "Unconfigure Live" {
            n162 = call "Unconfigure Live.vi"("error in (no error)"=w291, "Frame Grabber Data in"=w288) -> ("error out"=w289:errorcluster)  [unwired: 9 in]
          }
          frame "End Recording" {
            n163 = call "End Recording.vi"("error in (no error)"=w295, "Frame Grabber Data in"=w293) -> ("error out"=w292:errorcluster)  [unwired: 9 in]
          }
          frame "Stop Playback" {
            n164 = Unbundle By Name(w307) -> ("AVI Refnum"=w308:T19, "Refnums"=w298:T12)
            n165 = local read "Initial Recording Settings"() -> (w296:T6)
            n166 = call "IMAQ AVI2 Close"("error in (no error)"=w309, "AVI Refnum"=w308) -> ("error out"=w303:errorcluster)  [unwired: 9 in]
            n167 = local write "Playback"(FALSE ("Playback")) -> ()
            n168 = Unbundle By Name(w298) -> ("Recording Settings Refnum"=w297:refnum<vi>)
            n169 = call "Set Controls Enable or Disable State Data Recorder.vi"("error in (no error)"=w303, "Refnum State"=Enabled_State_Control."Wait", "Refnums In"=w298) -> ("error out"=w300:errorcluster)  [unwired: 8 in]
            n170 = Bundle By Name(cluster=w307, "AVI Refnum"=refnum<k0> refnum) -> (w306:T18)
            n171 = property class="Clust (strict)"(reference=w297, error in=w300, "Value"=w296) -> (error out=w299:errorcluster)  [unwired: 1 out]
          }
          frame "Error Handling" {
            # "just in case"
            n172 = call "End Recording.vi"("error in (no error)"=w316, "Frame Grabber Data in"=w311) -> ("error out"=w315:errorcluster)  [unwired: 9 in]
            n173 = call <vilib>:"Simple Error Handler.vi"("error in (no error)"=w315) -> ("error out"=w318:errorcluster)  [unwired: 4 in, 4 out]
            n174 = Unbundle By Name(w311) -> ("Refnums"=w310:T12)
            n175 = call <vilib>:"Clear Errors.vi"("error in (no error)"=w318) -> ("error out"=w314:errorcluster)  [unwired: 5 in, 1 out]
            n176 = call "Set Controls Enable or Disable State Data Recorder.vi"("error in (no error)"=w314, "Refnum State"=Enabled_State_Control."Wait", "Refnums In"=w310) -> ("error out"=w313:errorcluster)  [unwired: 8 in]
          }
          frame "Shutdown" {
            n177 = local read "Frame Grabber \nConnected?"() -> (w319:bool)
            n178 = call "Shutdown Frame Grabber.vi"("error in (no error)"=w324, "Frame grabber connected?"=w319, "Frame Grabber Data in"=w322) -> ("error out"=w323:errorcluster, "Disconnect"=w320:bool, "Frame Grabber Data out"=w321:T18)  [unwired: 6 in]
            n179 = local write "Frame Grabber \nConnected?"(w320) -> ()
          }
        }
        n180 = case shown="True" "Home" {
          tunnel: w117 -> [w129 w134]
          tunnel: w119 -> [w130 w133]
          tunnel: [w130 w132] -> w118
          tunnel: [w129 w131] -> w116
          frame False {
          }
          frame True {
            n181 = call "Create 3D Shapes.vi"("error in (no error)"=w133, "Frame Grabber Data In"=w134) -> ("error out"=w132:errorcluster, "Frame Grabber Data Out"=w131:T18)  [unwired: 8 in]
            n182 = Unbundle By Name(w131) -> ("Scene"=w135:refnum<vi>)
            n183 = local write "Probe Position"(w135) -> ()
          }
        }
        n184 = Select(t=Frame_Grabber_State."Error Handling", s=w118, f=w124) -> (s? t:f=w123:T22)
      }
      n185 = while {
        shift-right: [w57] -> w41
        shift-left: w43 -> [w59]
        shift-right: [w55] -> _
        shift-left: Optitrack_State."Init" ("OptiTrack State") -> [w60]
        tunnel: w32 -> [w58]
        shift-right: [w52] -> _
        shift-left: _ -> [w51]
        tunnel: w36 -> [w50]
        tunnel: w35 -> [w49]
        stop <- w53 stop-if-true
        # "Tracker State Machine"
        n186 = case shown="\"Init\"" w60 {
          tunnel: w59 -> [w66 w69 w93 w100 w107]
          tunnel: [w65 w73 w92 w98 w102] -> w57
          tunnel: w58 -> [w64 _ _ _ _]
          tunnel: [w63 Optitrack_State."Grab Rigid Body Data" ("OptiTrack State") w88 Optitrack_State."Wait" ("OptiTrack State") Optitrack_State."Wait" ("OptiTrack State")] -> w54
          tunnel: [_ _ _ _ TRUE] -> w53
          tunnel: [w62 w70 w87 w97 w105] -> w52
          tunnel: w51 -> [w62 _ w91 w97 w101]
          tunnel: w50 -> [_ w67 _ _ w103]
          tunnel: w49 -> [_ w68 _ _ _]
          frame "Wait", Default {
            n187 = Unbundle By Name(w64) -> ("Tracker State"=w61:refnum<queue>)
            n188 = Dequeue Element(queue=w61, error in (no error)=w66) -> (element=w63:T21, error out=w65:errorcluster)  [unwired: 1 in, 2 out]
          }
          frame "Init" {
            n189 = case shown="\"Aurora\"" w67 {
              tunnel: [w77 w82] -> w74
              tunnel: [w76 w81] -> w73
              tunnel: [w75 w80] -> w72
              tunnel: w69 -> [_ w79]
              tunnel: w68 -> [_ w78]
              frame "OptiTrack" {
                n190 = call "Init OptiTrack.vi"() -> ("error out"=w76:errorcluster, "OptiTrack Connected?"=w75:bool, "Frame Grabber Data"=w77:T26)  [unwired: 9 in]
              }
              frame "Aurora" {
                n191 = call "Init Aurora.vi"("error in (no error)"=w79, "Aurora COM Port"=w78) -> ("error out"=w81:errorcluster, "Aurora Connected?"=w80:bool, "Frame Grabber Data"=w82:T28)  [unwired: 7 in]
              }
            }
            "Tracker \nConnected?" <- w72
            n192 = Bundle By Name(cluster=w74, "Tracker"=w67) -> (w70:T28)
          }
          frame "Grab Rigid Body Data" {
            n193 = local read "Playback"() -> (w85:bool)
            n194 = call "Read Rigid Body Data.vi"("error in (no error)"=w93, "Tracking Data In"=w91) -> ("error out"=w92:errorcluster, "Tracking Data Out"=w87:T28)  [unwired: 8 in]
            n195 = Unbundle By Name(w87) -> ("Rigid Body Data"=w84:T1[])
            "Rigid Bodies" <- w84
            n196 = Index Array(array=w84) -> (element=w83:T1)  [unwired: 1 in]
            "Rigid Body" <- w83
            n197 = case shown="False" w85 {
              tunnel: w83 -> [w95 _]
              frame False {
                n198 = Unbundle By Name(w95) -> ("Tracked?"=→"Tracked?":bool)
              }
              frame True {
              }
            }
            n199 = Select(t=Optitrack_State."Shutdown" ("f"), s="stop", f=Optitrack_State."Grab Rigid Body Data" ("OptiTrack State")) -> (s? t:f=w88:T21)
          }
          frame "Error Handling" {
            n200 = call <vilib>:"Simple Error Handler.vi"("error in (no error)"=w100) -> ("error out"=w99:errorcluster)  [unwired: 4 in, 4 out]
            n201 = call <vilib>:"Clear Errors.vi"("error in (no error)"=w99) -> ("error out"=w98:errorcluster)  [unwired: 5 in, 1 out]
          }
          frame "Shutdown" {
            n202 = case shown="\"Aurora\"" w103 {
              tunnel: w107 -> [w111 w114]
              tunnel: [w110 w113] -> w102
              tunnel: w101 -> [w109 w112]
              frame "OptiTrack" {
                n203 = call "Close Motive and PacketClient.vi"("Error In"=w111, "OptiTrack Data"=w109) -> ("Error Out"=w110:errorcluster)  [unwired: 9 in]
              }
              frame "Aurora" {
                n204 = call "Close AuroraTracker.vi"("Error In"=w114, "OptiTrack Data"=w112) -> ("Error Out"=w113:errorcluster)  [unwired: 9 in]
              }
            }
            n205 = Bundle By Name(cluster=w101, "VISA resource name"=refnum<visa-resource-name> refnum) -> (w105:T28)
          }
        }
        n206 = Select(t=Optitrack_State."Error Handling" ("OptiTrack State"), s=w57, f=w54) -> (s? t:f=w55:T21)
      }
      n207 = Merge Errors(w48, w47, w41) -> (w46:errorcluster)
      n208 = call "Release Queues.vi"("error in (no error) in"=w46, "Queues"=w32) -> ("error out"=w45:errorcluster)  [unwired: 9 in]
      n209 = call <vilib>:"Simple Error Handler.vi"("error in (no error)"=w45) -> ("error out"=w38:errorcluster)  [unwired: 4 in, 4 out]
      "Initial Recording Settings" <- w25
    }
    frame True {
    }
  }
  n210 = call "Set Controls Enable or Disable State Data Recorder.vi"("error in (no error)"=w13, "Refnum State"=Enabled_State_Control."Shutdown", "Refnums In"=w7) -> ()  [unwired: 8 in, 1 out]
